vi "Close.vi"(8 "error in (no error)":errorcluster, 11 "MicronServer in":refnum<class "GRPCService.lvclass">) -> (0 "error out":errorcluster, 3 "MicronServer out":refnum<class "GRPCService.lvclass">)   [LabVIEW 2019, in "MicronGRPCServer.lvlib" / "GRPCService.lvclass"]
uses:
  GRPCService.lvclass
  GRPCService.lvclass/GRPCService.ctl
  Generated/MicronGRPCGeneratedServer/MicronGRPCGeneratedServer.lvlib
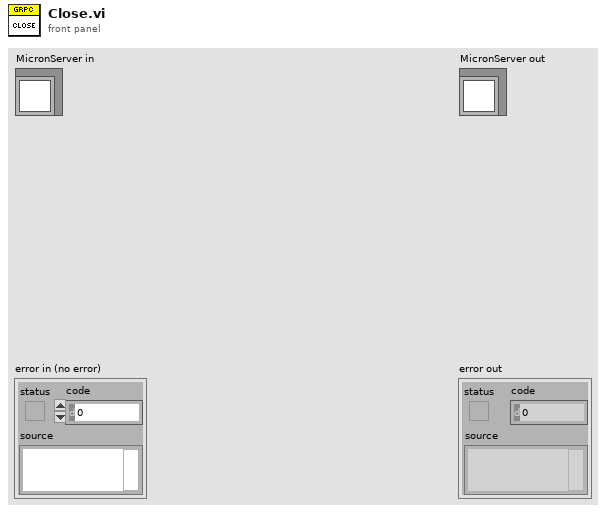
[diagram p1: front panel]
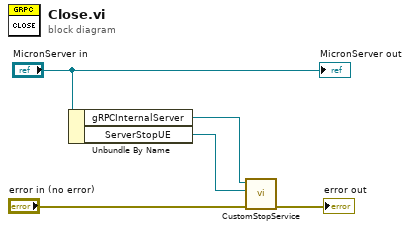
[diagram p0: block diagram]
diagram:
  n1 = Unbundle By Name("MicronServer in") -> ("gRPCInternalServer"=w2:refnum<class "Servicer.lvclass">, "ServerStopUE"=w1:refnum<user-event>)
  n2 = call "CustomStopService.vi"("error in (no error)"="error in (no error)", "Server Stop"=w1, "gRPC Server"=w2) -> ("error out"=→"error out":errorcluster)  [unwired: 8 in]
  "MicronServer out" <- "MicronServer in"
